vi "One Ball Hot.vi"() -> ()   [LabVIEW 2014]
uses:
  Team Code/Robot Global Data.vi
panel:
  out "Angle":dbl
  out "Distance (in)":dbl
  in  "Min. Power":dbl=0.1 format="%#_13g"
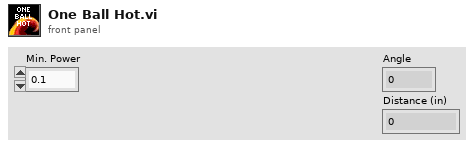
[diagram p1: front panel]
types:
  T1 = cluster{"FIRE!!!":bool, "Loader":bool, "Lock":bool, "Load":bool, "Pass":bool, "Grab":bool, "PANIC":bool, "Don't Cock":bool, "Roller Speed":dbl}
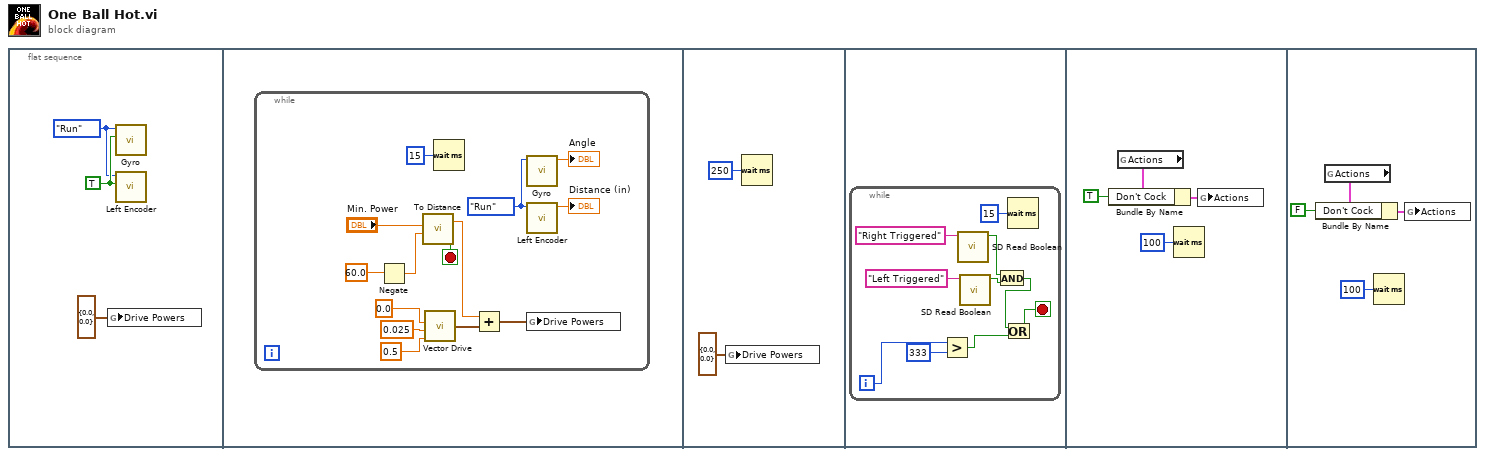
[diagram p0: block diagram]
diagram:
  n1 = flat-sequence {
    frame #0 {
      w2 = enum16{"Start", "Run", "End"}."Run" ("Enum")
      w3 = TRUE ("Reset")
      n2 = global write "Robot Global Data.vi" "Drive Powers"(cluster{"Right":dbl, "Left":dbl} {"Right"=0.0, "Left"=0.0} ("Drive Powers")) -> ()
      n3 = call "Gyro.vi"("Reset"=w3, "Enum"=w2) -> ()  [unwired: 9 in, 1 out]
      n4 = call "Left Encoder.vi"("Reset"=w3, "Enum"=w2) -> ()  [unwired: 8 in, 2 out]
    }
    frame #1 {
      n5 = while {
        stop <- w16 stop-if-true
        w9 = enum16{"Start", "Run", "End"}."Run" ("Enum")
        n6 = Negate(x=60.0) -> (-x=w7:dbl)
        n7 = call "To Distance.vi"("Destination Dist (in)"=w7, "Min. Power"="Min. Power") -> ("Reached Distance"=w16:bool, "Base Speed"=w6:dbl)  [unwired: 2 in]
        n8 = call "Vector Drive.vi"("Tolerance"=0.5, "Min. Power"=0.025, "Angle"=0.0) -> ("Motor Powers"=w12:cluster{"RMotor":dbl, "LMotor":dbl})  [unwired: 1 in]
        n9 = Wait (ms)(milliseconds to wait=u32 15) -> ()  [unwired: 1 out]
        n10 = Add(x=w6, y=w12) -> (x+y=w11:cluster{"RMotor":dbl, "LMotor":dbl})
        n11 = call "Gyro.vi"("Enum"=w9) -> ("Angle"=→"Angle":dbl)  [unwired: 10 in]
        n12 = call "Left Encoder.vi"("Enum"=w9) -> ("Distance (in)"=→"Distance (in)":dbl)  [unwired: 9 in, 1 out]
        n13 = global write "Robot Global Data.vi" "Drive Powers"(w11) -> ()
      }
    }
    frame #2 {
      n14 = global write "Robot Global Data.vi" "Drive Powers"(cluster{"Right":dbl, "Left":dbl} {"Right"=0.0, "Left"=0.0} ("Drive Powers")) -> ()
      n15 = Wait (ms)(milliseconds to wait=u32 250) -> ()  [unwired: 1 out]
    }
    frame #3 {
      n16 = while {
        i -> [w22]
        stop <- w24 stop-if-true
        n17 = Greater?(x=w22, y=333) -> (0:w20:bool)
        n18 = call <vilib>:"SD Read Boolean.vi"("Name"="Right Triggered") -> ("Boolean"=w25:bool)  [unwired: 8 in, 2 out]
        n19 = call <vilib>:"SD Read Boolean.vi"("Name"="Left Triggered") -> ("Boolean"=w26:bool)  [unwired: 8 in, 2 out]
        n20 = And(x=w25, y=w26) -> (x .and. y?=w23:bool)
        n21 = Or(x=w23, y=w20) -> (x .or. y?=w24:bool)
        n22 = Wait (ms)(milliseconds to wait=u32 15) -> ()  [unwired: 1 out]
      }
    }
    frame #4 {
      n23 = global read "Robot Global Data.vi" "Actions"() -> (w32:T1)
      n24 = Bundle By Name(cluster=w32, "Don't Cock"=TRUE ("Primary Action")) -> (w33:T1)
      n25 = Wait (ms)(milliseconds to wait=u32 100) -> ()  [unwired: 1 out]
      n26 = global write "Robot Global Data.vi" "Actions"(w33) -> ()
    }
    frame #5 {
      n27 = global read "Robot Global Data.vi" "Actions"() -> (w36:T1)
      n28 = Bundle By Name(cluster=w36, "Don't Cock"=FALSE ("Primary Action")) -> (w35:T1)
      n29 = Wait (ms)(milliseconds to wait=u32 100) -> ()  [unwired: 1 out]
      n30 = global write "Robot Global Data.vi" "Actions"(w35) -> ()
    }
  }
